vi "Destroy.vi"(8 "Error In":errorcluster, 11 "Render":refnum<class "Render.lvclass">) -> (0 "Error Out":errorcluster, 3 "Reader":refnum<class "Abstract.lvclass">)   [LabVIEW 2018]
uses:
  Render.lvclass
  Readers/Abstract/Abstract.lvclass
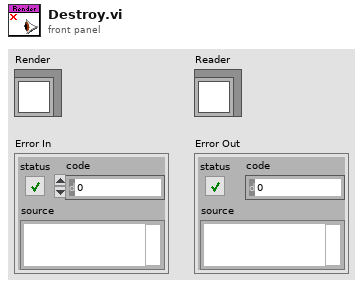
[diagram p1: front panel]
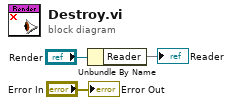
[diagram p0: block diagram]
diagram:
  n1 = Unbundle By Name("Render") -> ("Reader"=→"Reader")
  "Error Out" <- "Error In"
